vi "ble_config_bonding.vi"(8 "error in (no error)":errorcluster, 10 "bondable?(F)":bool, 11 "COM Bluegiga in":refnum<visa-resource-name>) -> (0 "error out":errorcluster, 3 "COM Bluegiga out":refnum<visa-resource-name>)   [LabVIEW 2013]
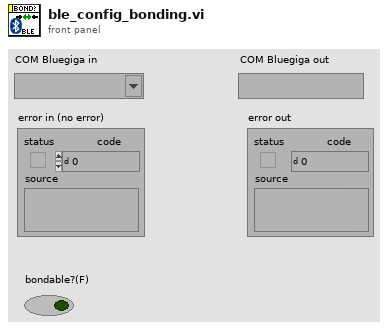
[diagram p1: front panel]
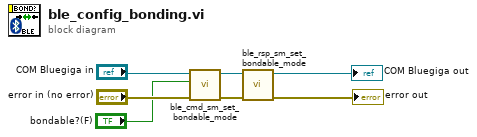
[diagram p0: block diagram]
diagram:
  n1 = call "ble_cmd_sm_set_bondable_mode.vi"("error in (no error)"="error in (no error)", "bondable?"="bondable?(F)", "COM Bluegiga in"="COM Bluegiga in") -> ("error out"=w7:errorcluster, "COM Bluegiga out"=w6:refnum<visa-resource-name>)  [unwired: 7 in]
  n2 = call "ble_rsp_sm_set_bondable_mode.vi"("error in (no error)"=w7, "COM Bluegiga in"=w6) -> ("error out"=→"error out":errorcluster, "COM Bluegiga out"=→"COM Bluegiga out":refnum<visa-resource-name>)  [unwired: 8 in]
